vi "FTW-Router-Construct.vi"(5 "Incoming Message Router Address":string="tcp://127.0.0.1:*", 11 "error in":errorcluster) -> (4 "FTW Router":refnum<class "FTW-Router.lvclass">, 6 "Inbox Address":string, 8 "Incoming Message":refnum<event-registration>, 15 "error out":errorcluster)   [LabVIEW 2013, in "FTW-Router.lvclass"]
uses:
  FTW-Router.lvclass
  message/FTW-Message.lvclass
  FTW-Router.lvclass/FTW-Router.ctl
  error/FTW-ERR-ThrowGenericError.vi
  error/FTW-ERR-ThrowError.vi
  error/FTW-ERR-NoErrorConstant.vi
  error/FTW-ERR-CallChain.vi
  string/FTW-STR-ReplaceWhitespace.vi
  socket/FTW-Socket.lvclass
panel:
  # "Inputs"
  # "Outputs"
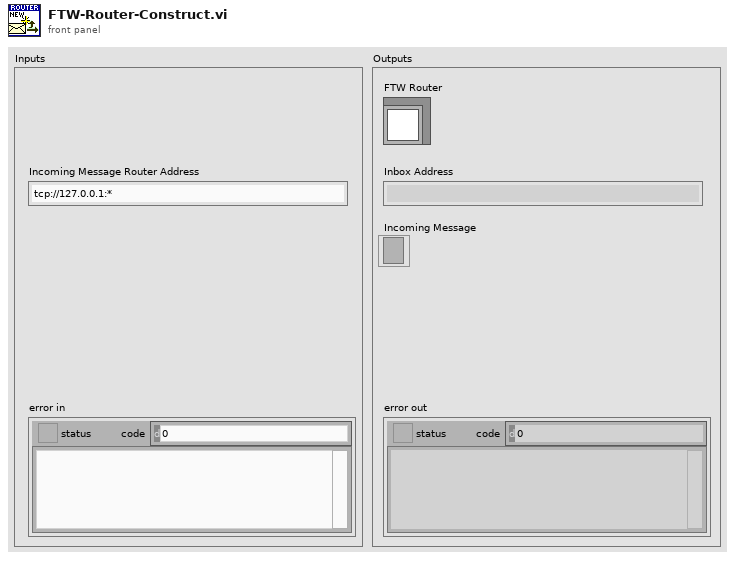
[diagram p1: front panel]
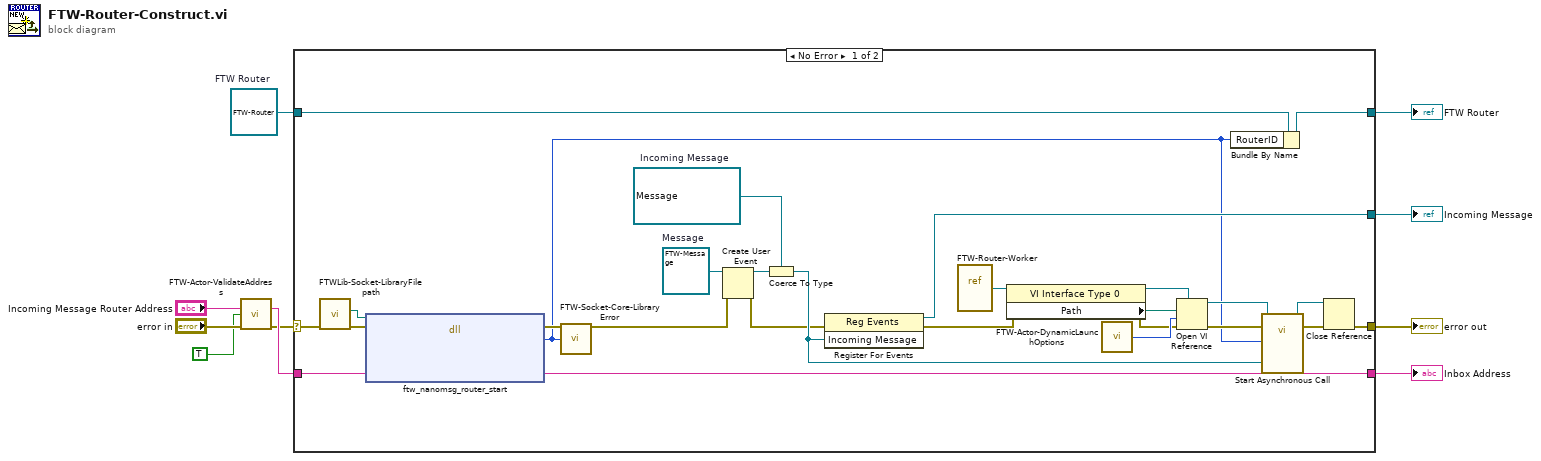
[diagram p0: block diagram]
diagram:
  w8 = refnum<class "FTW-Router.lvclass"> refnum  # FTW Router
  n1 = call "FTW-Actor-ValidateAddress.vi"("Address"="Incoming Message Router Address", "Allow wildcard replacement?"=TRUE, "error in"="error in") -> ("Sanitized Address"=w5:string, "error out"=w3:errorcluster)  [unwired: 10 in, 1 out]
  n2 = case shown="No Error" w3 {
    selector: w3 -> [w17 w40]
    tunnel: [w36 w39] -> w10
    tunnel: [w14 w40] -> w9
    tunnel: w8 -> [w37 w39]
    tunnel: w5 -> [w18 w38]
    tunnel: [w13 _] -> w1
    tunnel: [w35 w38] -> w7
    frame No Error {
      w11 = refnum<class "FTW-Message.lvclass"> refnum  # Message
      w30 = refnum<user-event> refnum  # Incoming Message
      n3 = call "FTWLib-Socket-LibraryFilepath.vi"("error in"=w17) -> ("error out"=w19:errorcluster, "Library Filepath"=w20:path)  [unwired: 8 in, 1 out]
      n4 = dll-call lib="?" fn="ftw_nanomsg_router_start"(path in=w20, error in=w19, "Address"=w18) -> (error out=w16:errorcluster, "Return Value"=w12:i64, "Address"=w35:string)  [unwired: 3 in, 1 out]
      n5 = call "FTW-Socket-Core-LibraryError.vi"("error in"=w16, "Return Value"=w12) -> ("error out"=w15:errorcluster)  [unwired: 13 in]
      n6 = Create User Event(user event datatype=w11, error in=w15) -> (user event=w29:refnum<user-event>, error out=w28:errorcluster)
      n7 = Coerce To Type(0:w29, 1:w30) -> (2:w34:refnum<user-event>)
      n8 = register-events(error in=w28, w34) -> (reference out=w13:refnum<event-registration>, error out=w31:errorcluster)  [unwired: 1 in]
      n9 = vi-ref "FTW-Router-Worker.vi"() -> (w21:refnum<vi>)
      n10 = property class="VI Interface Type 0"(reference=w21, error in=w31) -> (reference out=w22:refnum<vi>, error out=w25:errorcluster, "Path"=w23:path)
      n11 = call "FTW-Actor-DynamicLaunchOptions.vi"() -> ("Open VI Ref Options"=w26:i32)  [unwired: 1 in]
      n12 = Open VI Reference(type specifier VI Refnum (for type only)=w22, vi path=w23, options=w26, error in (no error)=w25) -> (vi reference=w27:refnum<vi>, error out=w24:errorcluster)  [unwired: 2 in]
      n13 = Bundle By Name(cluster=w37, "RouterID"=w12) -> (w36:refnum<class "FTW-Router.lvclass">)
      n14 = call-by-ref "Start Asynchronous Call"(reference=w27, error in=w24, "Backend Handler"=w34, "RouterID"=w12) -> (reference out=w32:refnum<vi>, error out=w33:errorcluster)  [unwired: 1 in]
      n15 = Close Reference(reference=w32, error in (no error)=w33) -> (error out=w14:errorcluster)
    }
    frame Error {
    }
  }
  "error out" <- w9
  "FTW Router" <- w10
  "Inbox Address" <- w7
  "Incoming Message" <- w1
